vi "libtiff3 calc Strip-mod.vi"(8 "error in (no error)":errorcluster, 11 "ImageIn":T3) -> (0 "error out":errorcluster, 1 "LastStrip":T1, 2 "Strip":T2, 3 "ImageOut":T3, 5 "NumberOfStrips":i32)   [LabVIEW 2020]
doc: "SciScan 1.0 151216\nCalculate the strip number and size for writing a striped TIFF"
uses:
  <vilib>/vision/Image Controls.llb/IMAQ Image.ctl
panel:
  out "Last sripSize in pixels":i32
  out "StripSize in pixels":i32
  out "LastStripRows":i32
  out "LastStripSize in bytes":i32
  out "StripSize in bytes":i32
  out "RowsPerStrip":u32
  out "RowSize in bits":u32
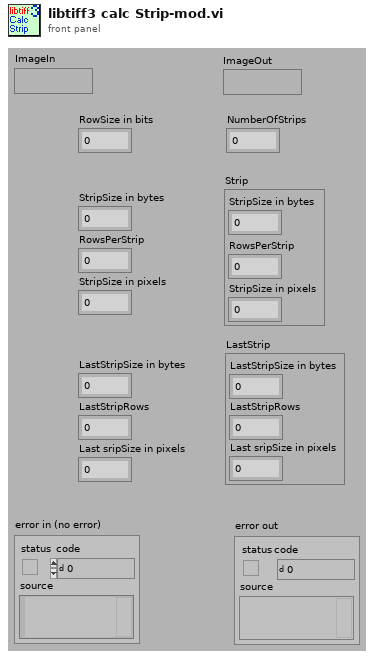
[diagram p1: front panel]
types:
  T1 = cluster{"LastStripSize in bytes":i32, "LastStripRows":i32, "Last sripSize in pixels":i32}
  T2 = cluster{"StripSize in bytes":i32, "RowsPerStrip":u32, "StripSize in pixels":i32}
  T3 = typedef "IMAQ Image.ctl" = refnum<image>
  T4 = typedef "Image Type" = u32
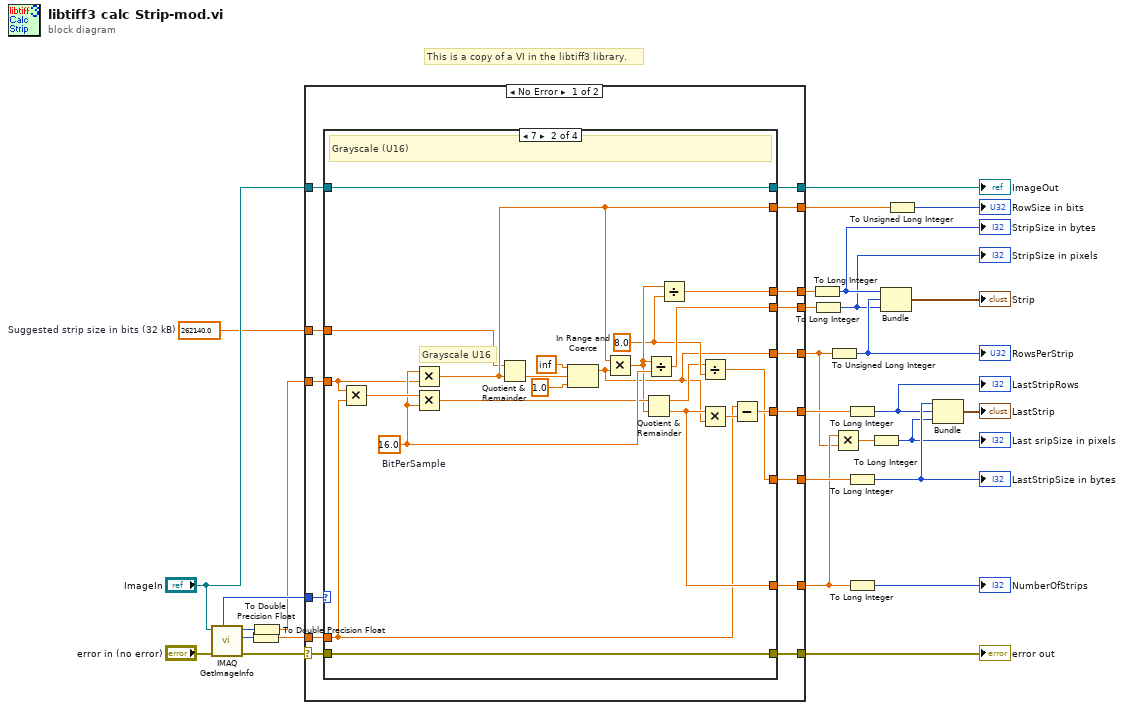
[diagram p0: block diagram]
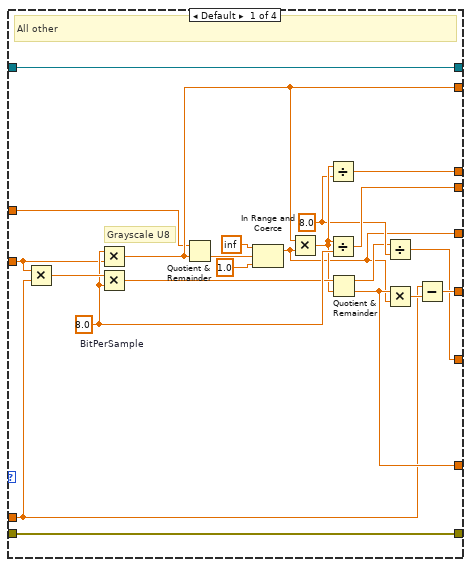
[diagram p2: hidden frame]
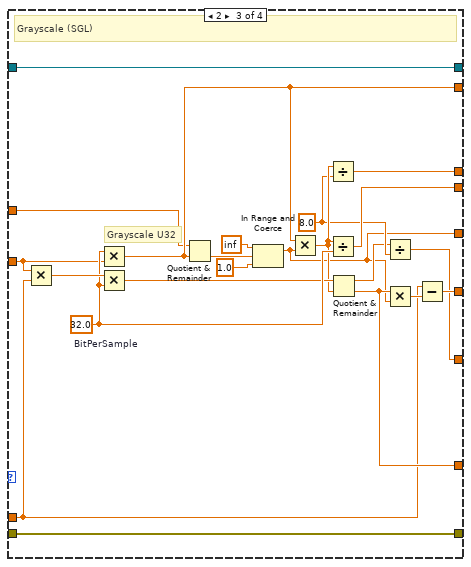
[diagram p3: hidden frame]
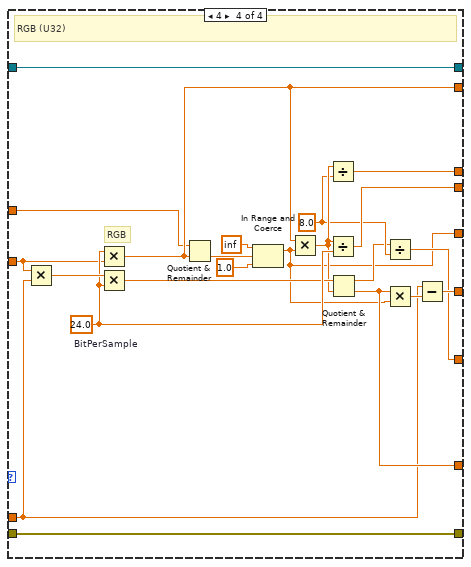
[diagram p4: hidden frame]
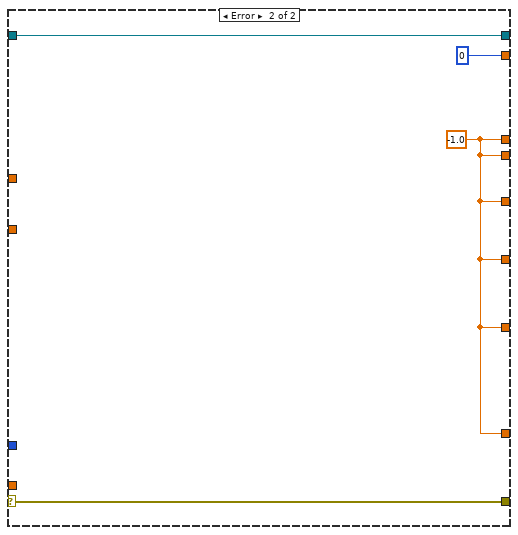
[diagram p5: hidden frame]
diagram:
  w14 = 262140.0  # Suggested strip size in bits (32 kB)
  # "This is a copy of a VI in the libtiff3 library."
  n1 = call "IMAQ GetImageInfo"("error in (no error)"="error in (no error)", "Image"="ImageIn") -> ("error out"=w25:errorcluster, "Y Resolution"=w16:i32, "X Resolution"=w15:i32, "Image Type"=w28:T4)  [unwired: 2 in, 4 out]
  n2 = To Double Precision Float(number=w16) -> (double precision float=w11:dbl)
  n3 = To Double Precision Float(number=w15) -> (double precision float=w12:dbl)
  n4 = case shown="No Error" w25 {
    selector: w25 -> [w35 w136]
    tunnel: [w44 u32 0] -> w29
    tunnel: [w43 w134] -> w13
    tunnel: [w42 w134] -> w6
    tunnel: [w41 w134] -> w21
    tunnel: [w40 w134] -> w17
    tunnel: [w39 w134] -> w19
    tunnel: [w38 w134] -> w22
    tunnel: w28 -> [w37 _]
    tunnel: "ImageIn" -> [w36 w135]
    tunnel: [w32 w136] -> w24
    tunnel: w12 -> [w34 _]
    tunnel: w11 -> [w33 _]
    tunnel: [w31 w135] -> w23
    tunnel: w14 -> [w30 _]
    frame No Error {
      n5 = case shown="7" w37 {
        tunnel: w35 -> [w56 w78 w100 w122]
        tunnel: [w65 w87 w109 w131] -> w44
        tunnel: [w63 w85 w107 w129] -> w43
        tunnel: [w45 w67 w89 w112] -> w42
        tunnel: [w61 w83 w105 w127] -> w41
        tunnel: [w53 w75 w97 w111] -> w40
        tunnel: [w59 w81 w103 w125] -> w39
        tunnel: [w50 w72 w94 w113] -> w38
        tunnel: w36 -> [w55 w77 w99 w121]
        tunnel: w34 -> [w58 w80 w102 w124]
        tunnel: w33 -> [w57 w79 w101 w123]
        tunnel: [w56 w78 w100 w122] -> w32
        tunnel: [w55 w77 w99 w121] -> w31
        tunnel: w30 -> [w49 w71 w93 w117]
        frame Default {
          w52 = 8.0 ("y")
          w62 = 8.0  # BitPerSample
          # "Grayscale U8"
          # "All other"
          n6 = Multiply(x=w58, y=w57) -> (x*y=w66:dbl)
          n7 = Multiply(x=w62, y=w58) -> (x*y=w65:dbl)
          n8 = Multiply(x=w66, y=w62) -> (x*y=w60:dbl)
          n9 = Quotient & Remainder(x=w49, y=w65) -> (floor(x/y)=w46:dbl)  [unwired: 1 out]
          n10 = In Range and Coerce(upper limit=inf, x=w46, lower limit=1.0) -> (coerced(x)=w45:dbl)  [unwired: 1 out]
          n11 = Multiply(x=w65, y=w45) -> (x*y=w54:dbl)
          n12 = Divide(x=w54, y=w52) -> (x/y=w53:dbl)
          n13 = Divide(x=w54, y=w62) -> (x/y=w61:dbl)
          n14 = Quotient & Remainder(x=w60, y=w54) -> (x-y*floor(x/y)=w51:dbl, floor(x/y)=w59:dbl)
          n15 = Divide(x=w51, y=w52) -> (x/y=w50:dbl)
          n16 = Multiply(x=w59, y=w45) -> (x*y=w64:dbl)
          n17 = Subtract(x=w57, y=w64) -> (x-y=w63:dbl)
        }
        frame 7 {
          w74 = 8.0 ("y")
          w84 = 16.0  # BitPerSample
          # "Grayscale U16"
          # "Grayscale (U16)"
          n18 = Multiply(x=w80, y=w79) -> (x*y=w88:dbl)
          n19 = Multiply(x=w84, y=w80) -> (x*y=w87:dbl)
          n20 = Multiply(x=w88, y=w84) -> (x*y=w82:dbl)
          n21 = Quotient & Remainder(x=w71, y=w87) -> (floor(x/y)=w68:dbl)  [unwired: 1 out]
          n22 = In Range and Coerce(upper limit=inf, x=w68, lower limit=1.0) -> (coerced(x)=w67:dbl)  [unwired: 1 out]
          n23 = Multiply(x=w87, y=w67) -> (x*y=w76:dbl)
          n24 = Quotient & Remainder(x=w82, y=w76) -> (x-y*floor(x/y)=w73:dbl, floor(x/y)=w81:dbl)
          n25 = Divide(x=w76, y=w84) -> (x/y=w83:dbl)
          n26 = Divide(x=w76, y=w74) -> (x/y=w75:dbl)
          n27 = Divide(x=w73, y=w74) -> (x/y=w72:dbl)
          n28 = Multiply(x=w81, y=w67) -> (x*y=w86:dbl)
          n29 = Subtract(x=w79, y=w86) -> (x-y=w85:dbl)
        }
        frame 2 {
          w96 = 8.0 ("y")
          w106 = 32.0  # BitPerSample
          # "Grayscale U32"
          # "Grayscale (SGL)"
          n30 = Multiply(x=w102, y=w101) -> (x*y=w110:dbl)
          n31 = Multiply(x=w106, y=w102) -> (x*y=w109:dbl)
          n32 = Multiply(x=w110, y=w106) -> (x*y=w104:dbl)
          n33 = Quotient & Remainder(x=w93, y=w109) -> (floor(x/y)=w90:dbl)  [unwired: 1 out]
          n34 = In Range and Coerce(upper limit=inf, x=w90, lower limit=1.0) -> (coerced(x)=w89:dbl)  [unwired: 1 out]
          n35 = Multiply(x=w109, y=w89) -> (x*y=w98:dbl)
          n36 = Divide(x=w98, y=w96) -> (x/y=w97:dbl)
          n37 = Divide(x=w98, y=w106) -> (x/y=w105:dbl)
          n38 = Quotient & Remainder(x=w104, y=w98) -> (x-y*floor(x/y)=w95:dbl, floor(x/y)=w103:dbl)
          n39 = Divide(x=w95, y=w96) -> (x/y=w94:dbl)
          n40 = Multiply(x=w103, y=w89) -> (x*y=w108:dbl)
          n41 = Subtract(x=w101, y=w108) -> (x-y=w107:dbl)
        }
        frame 4 {
          w119 = 8.0 ("y")
          w128 = 24.0  # BitPerSample
          # "RGB"
          # "RGB (U32)"
          n42 = Multiply(x=w124, y=w123) -> (x*y=w132:dbl)
          n43 = Multiply(x=w128, y=w124) -> (x*y=w131:dbl)
          n44 = Multiply(x=w132, y=w128) -> (x*y=w126:dbl)
          n45 = Quotient & Remainder(x=w117, y=w131) -> (floor(x/y)=w114:dbl)  [unwired: 1 out]
          n46 = In Range and Coerce(upper limit=inf, x=w114, lower limit=1.0) -> (coerced(x)=w112:dbl)  [unwired: 1 out]
          n47 = Multiply(x=w131, y=w112) -> (x*y=w120:dbl)
          n48 = Divide(x=w120, y=w119) -> (x/y=w111:dbl)
          n49 = Divide(x=w120, y=w128) -> (x/y=w127:dbl)
          n50 = Quotient & Remainder(x=w126, y=w120) -> (x-y*floor(x/y)=w118:dbl, floor(x/y)=w125:dbl)
          n51 = Divide(x=w118, y=w119) -> (x/y=w113:dbl)
          n52 = Multiply(x=w125, y=w112) -> (x*y=w130:dbl)
          n53 = Subtract(x=w123, y=w130) -> (x-y=w129:dbl)
        }
      }
    }
    frame Error {
      w134 = -1.0
    }
  }
  "error out" <- w24
  "ImageOut" <- w23
  n54 = To Long Integer(number=w17) -> (32bit integer=w7:i32)
  "StripSize in bytes" <- w7
  n55 = To Long Integer(number=w21) -> (32bit integer=w4:i32)
  "StripSize in pixels" <- w4
  n56 = To Unsigned Long Integer(number=w6) -> (unsigned 32bit integer=w5:u32)
  "RowsPerStrip" <- w5
  n57 = Multiply(x=w19, y=w6) -> (x*y=w9:dbl)
  n58 = To Long Integer(number=w13) -> (32bit integer=w2:i32)
  "LastStripRows" <- w2
  n59 = To Long Integer(number=w22) -> (32bit integer=w3:i32)
  "LastStripSize in bytes" <- w3
  n60 = To Long Integer(number=w19) -> (32bit integer=→"NumberOfStrips":i32)
  n61 = To Long Integer(number=w9) -> (32bit integer=w1:i32)
  "Last sripSize in pixels" <- w1
  n62 = Bundle(w7, w5, w4) -> (→"Strip":cluster{i32, u32, i32})  [unwired: 1 in]
  n63 = To Unsigned Long Integer(number=w29) -> (unsigned 32bit integer=→"RowSize in bits":u32)
  n64 = Bundle(w3, w2, w1) -> (→"LastStrip":cluster{i32, i32, i32})  [unwired: 1 in]
